vi "MGCC_FntStaMach_Initialization.vi"() -> (0 "error out":errorcluster)   [LabVIEW 2016]
doc: "This VI is used to initize the events and flags in the FSM. In the future, it may be used to initize the variables in other function VIs."
uses:
  <vilib>/Utility/error.llb/Error Cluster From Error Code.vi
  MGCC_FntStaMach_gobal.vi
  <vilib>/ErrorRing/Error Ring.xnode
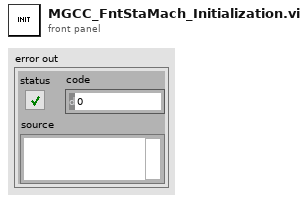
[diagram p1: front panel]
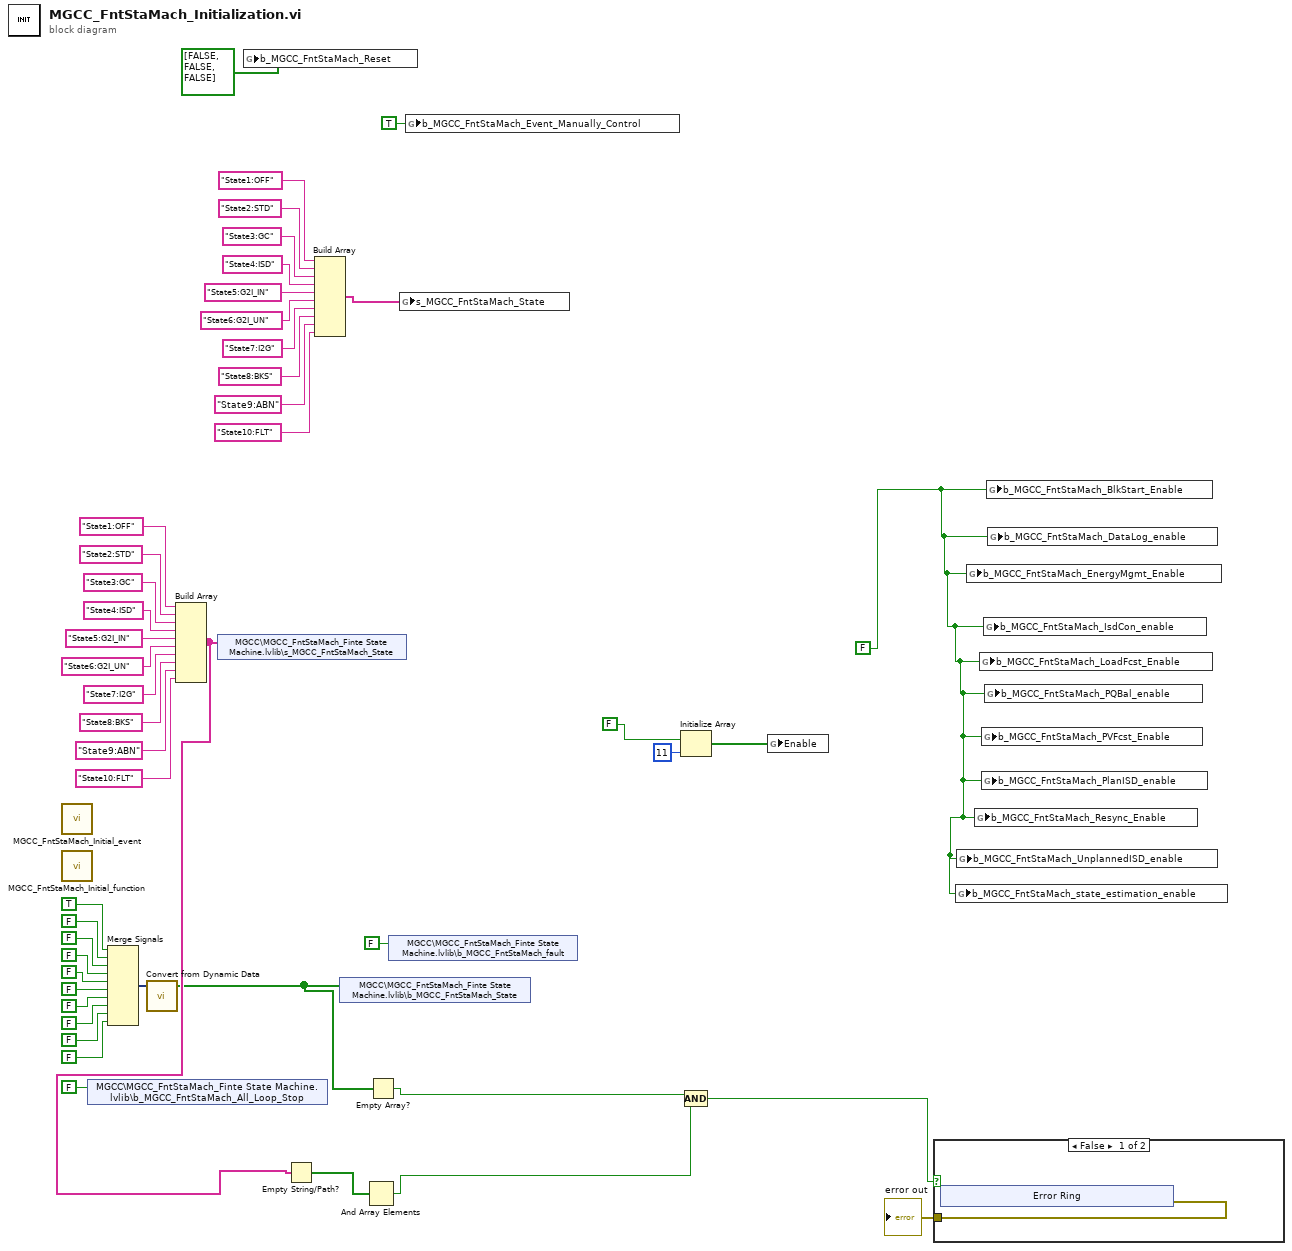
[diagram p0: block diagram]
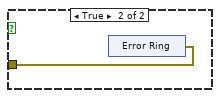
[diagram p2: hidden frame]
diagram:
  w15 = FALSE
  n1 = call "MGCC_FntStaMach_Initial_event.vi"() -> ()  [unwired: 12 in]
  n2 = call "MGCC_FntStaMach_Initial_function.vi"() -> ()  [unwired: 12 in]
  n3 = shared-variable "MGCC\\MGCC_FntStaMach_Finte State Machine.lvlib\\b_MGCC_FntStaMach_All_Loop_Stop"(FALSE ("ALL loop stop")) -> ()  [unwired: 1 in, 1 out]
  n4 = Merge Signals(TRUE ("State3"), FALSE ("State3"), FALSE ("State3"), FALSE ("State3"), FALSE ("State3"), FALSE ("State3"), FALSE ("State3"), FALSE ("State3"), FALSE ("State3"), FALSE ("State3")) -> (w37:dynamicdata)
  n5 = call "Convert from Dynamic Data"("Dynamic Data Type"=w37) -> ("Array"=w21:bool[])  [unwired: 3 in]
  n6 = Build Array("State1:OFF", "State2:STD", "State3:GC", "State4:ISD", "State5:G2I_IN", "State6:G2I_UN", "State7:I2G", "State8:BKS", "State9:ABN", "State10:FLT") -> (w23:string[])
  n7 = shared-variable "MGCC\\MGCC_FntStaMach_Finte State Machine.lvlib\\s_MGCC_FntStaMach_State"(w23) -> ()  [unwired: 1 in, 1 out]
  n8 = global write "MGCC_FntStaMach_gobal.vi" "b_MGCC_FntStaMach_Reset"(bool[] [FALSE, FALSE, FALSE] ("b_MGCC_FntStaMach_Reset")) -> ()
  n9 = Empty String/Path?(string/path=w23) -> (empty?=w22:bool[])
  n10 = Build Array("State1:OFF", "State2:STD", "State3:GC", "State4:ISD", "State5:G2I_IN", "State6:G2I_UN", "State7:I2G", "State8:BKS", "State9:ABN", "State10:FLT") -> (w2:string[])
  n11 = shared-variable "MGCC\\MGCC_FntStaMach_Finte State Machine.lvlib\\b_MGCC_FntStaMach_State"(w21) -> ()  [unwired: 1 in, 1 out]
  n12 = And Array Elements(Boolean array=w22) -> (logical AND=w24:bool)
  n13 = Empty Array?(array=w21) -> (empty?=w20:bool)
  n14 = shared-variable "MGCC\\MGCC_FntStaMach_Finte State Machine.lvlib\\b_MGCC_FntStaMach_fault"(FALSE ("b_MGCC_FntStaMach_fault")) -> ()  [unwired: 1 in, 1 out]
  n15 = global write "MGCC_FntStaMach_gobal.vi" "s_MGCC_FntStaMach_State"(w2) -> ()
  n16 = global write "MGCC_FntStaMach_gobal.vi" "b_MGCC_FntStaMach_Event_Manually_Control"(TRUE ("b_MGCC_FntStaMach_Event_Manually_Control")) -> ()
  n17 = Initialize Array(FALSE, 11 ("dimension size")) -> (w16:bool[])
  n18 = Compound Arithmetic op=AND(w20, w24) -> (w19:bool)
  n19 = global write "MGCC_FntStaMach_gobal.vi" "Enable"(w16) -> ()
  n20 = case shown="False" w19 {
    tunnel: [w48 w54] -> w1
    frame False {
      n21 = xnode "Error Ring"() -> ("error out"=w48:errorcluster)
    }
    frame True {
      n22 = xnode "Error Ring"() -> ("error out"=w54:errorcluster)
    }
  }
  "error out" <- w1
  n23 = global write "MGCC_FntStaMach_gobal.vi" "b_MGCC_FntStaMach_state_estimation_enable"(w15) -> ()
  n24 = global write "MGCC_FntStaMach_gobal.vi" "b_MGCC_FntStaMach_UnplannedISD_enable"(w15) -> ()
  n25 = global write "MGCC_FntStaMach_gobal.vi" "b_MGCC_FntStaMach_EnergyMgmt_Enable"(w15) -> ()
  n26 = global write "MGCC_FntStaMach_gobal.vi" "b_MGCC_FntStaMach_Resync_Enable"(w15) -> ()
  n27 = global write "MGCC_FntStaMach_gobal.vi" "b_MGCC_FntStaMach_LoadFcst_Enable"(w15) -> ()
  n28 = global write "MGCC_FntStaMach_gobal.vi" "b_MGCC_FntStaMach_PVFcst_Enable"(w15) -> ()
  n29 = global write "MGCC_FntStaMach_gobal.vi" "b_MGCC_FntStaMach_PlanISD_enable"(w15) -> ()
  n30 = global write "MGCC_FntStaMach_gobal.vi" "b_MGCC_FntStaMach_IsdCon_enable"(w15) -> ()
  n31 = global write "MGCC_FntStaMach_gobal.vi" "b_MGCC_FntStaMach_PQBal_enable"(w15) -> ()
  n32 = global write "MGCC_FntStaMach_gobal.vi" "b_MGCC_FntStaMach_BlkStart_Enable"(w15) -> ()
  n33 = global write "MGCC_FntStaMach_gobal.vi" "b_MGCC_FntStaMach_DataLog_enable"(w15) -> ()
